vi "DAQmx Timing (Implicit).vi"(0 "task/channels in":refnum<k21>, 1 "sample mode":i32(ring)=10178 items=["Finite Samples"=10178, "Continuous Samples"=10123, "Hardware Timed Single Point"=12522], 2 "samples per channel":i32=1000, 11 "error in":errorcluster) -> (4 "task out":refnum<k21>, 15 "error out":errorcluster)   [LabVIEW 2011]
doc: "Sets only the number of samples to acquire or generate without specifying timing. Typically, you should use this instance when the task does not require sample timing, such as tasks that use counters for buffered frequency measurement, buffered period measurement, or pulse train generation. For finite counter output tasks, <B>samples per channel</B> is the number of pulses to generate."
uses:
  C:/Program Files/National Instruments/LabVIEW 2011/resource/objmgr/daqmx.rc
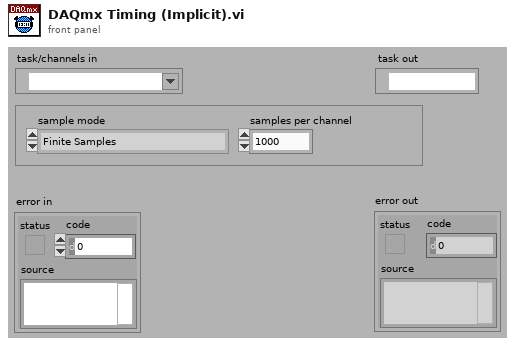
[diagram p1: front panel]
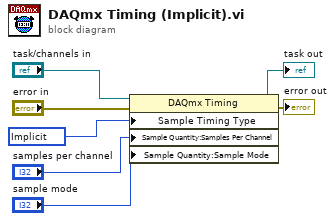
[diagram p0: block diagram]
diagram:
  w1 = 10451 items=["Sample Clock"=10388, "Handshake"=10389, "Implicit"=10451, "On Demand"=10390, "Change Detection"=12504] ("Sample Timing Type")
  n1 = property class="DAQmx Timing"(reference="task/channels in", error in="error in", "Sample Timing Type"=w1, "Sample Quantity:Samples Per Channel"="samples per channel", "Sample Quantity:Sample Mode"="sample mode") -> (reference out=→"task out":refnum<k21>, error out=→"error out":errorcluster)
